vi "ValueAsBase64.vi"(8 "error in (no error)":errorcluster, 11 "Parameter":string="  <value><base64>YWJjZA==</base64></value>\n    ") -> (0 "error out":errorcluster, 3 "value":string)   [LabVIEW 2009]
doc: "Convert XML-RPC base64 value to binary string"
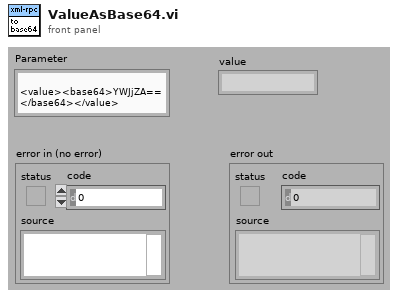
[diagram p1: front panel]
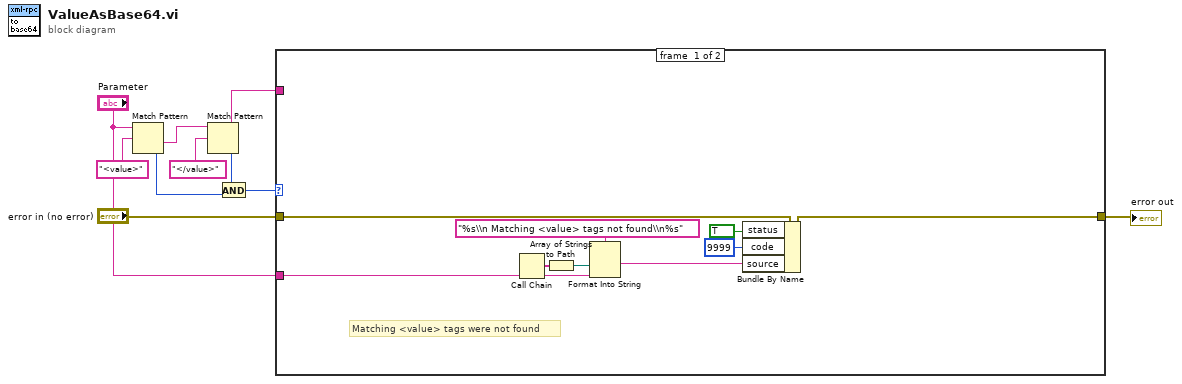
[diagram p0: block diagram]
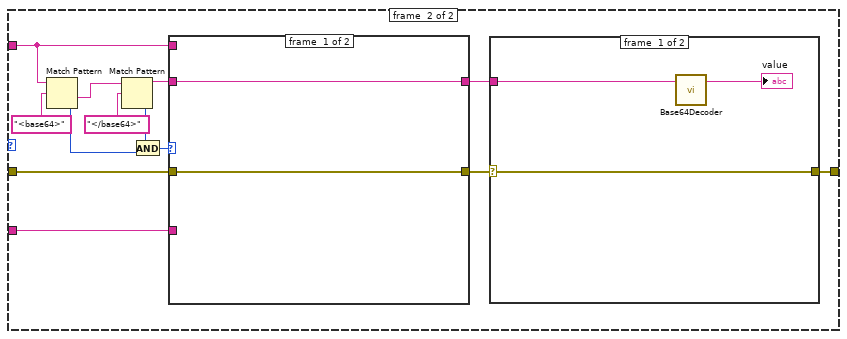
[diagram p2: hidden frame]
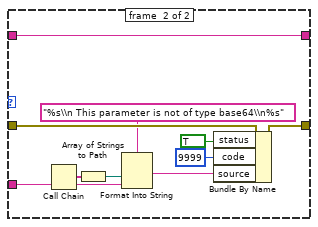
[diagram p4: hidden frame]
diagram:
  n1 = Match Pattern(string="Parameter", regular expression="<value>") -> (after substring=w9:string, offset past match=w2:i32)  [unwired: 1 in, 2 out]
  n2 = Match Pattern(string=w9, regular expression="</value>") -> (before substring=w7:string, offset past match=w3:i32)  [unwired: 1 in, 2 out]
  n3 = And(x=w3, y=w2) -> (x .and. y?=w1:i32)
  n4 = case shown="Default" w1 {
    tunnel: w7 -> [_ w29]
    tunnel: "error in (no error)" -> [w13 w27]
    tunnel: [w12 w22] -> w5
    tunnel: "Parameter" -> [w16 w26]
    frame #0 {
      # "Matching <value> tags were not found"
      n5 = Call Chain() -> (call chain=w19:string[])
      n6 = Array of Strings to Path(0:w19) -> (2:w18:path)  [unwired: 1 in]
      n7 = Format Into String(format string="%s\\n Matching <value> tags not found\\n%s", w18, w16) -> (resulting string=w11:string)  [unwired: 2 in, 1 out]
      n8 = Bundle By Name(cluster=w13, "status"=TRUE, "code"=9999, "source"=w11) -> (w12:errorcluster)
    }
    frame #1 {
      n9 = Match Pattern(string=w29, regular expression="<base64>") -> (after substring=w31:string, offset past match=w24:i32)  [unwired: 1 in, 2 out]
      n10 = Match Pattern(string=w31, regular expression="</base64>") -> (before substring=w28:string, offset past match=w25:i32)  [unwired: 1 in, 2 out]
      n11 = And(x=w25, y=w24) -> (x .and. y?=w23:i32)
      n12 = case shown="-1" w23 {
        tunnel: w29 -> [_ _]
        tunnel: w28 -> [w38 w39]
        tunnel: [w38 w39] -> w21
        tunnel: w27 -> [w37 w48]
        tunnel: [w37 w47] -> w20
        tunnel: w26 -> [_ w46]
        frame #0 {
        }
        frame #1 {
          n13 = Call Chain() -> (call chain=w45:string[])
          n14 = Array of Strings to Path(0:w45) -> (2:w42:path)  [unwired: 1 in]
          n15 = Format Into String(format string="%s\\n This parameter is not of type base64\\n%s", w42, w46) -> (resulting string=w41:string)  [unwired: 2 in, 1 out]
          n16 = Bundle By Name(cluster=w48, "status"=TRUE, "code"=9999, "source"=w41) -> (w47:errorcluster)
        }
      }
      n17 = case shown="No Error" w20 {
        selector: w20 -> [w35 w36]
        tunnel: [w35 w36] -> w22
        tunnel: w21 -> [w34 _]
        frame #0 {
          n18 = call "Base64Decoder.vi"("String In"=w34) -> ("String Out"=→"value":string)  [unwired: 9 in, 1 out]
        }
        frame #1 {
          # "don't try to convert if we can't find a valid tag"
        }
      }
    }
  }
  "error out" <- w5
